vi "Choreo_Trajectory_GetTrajState.vi"(9 "index":i32, 11 "ChoreoTrajectory":T2) -> (3 "ChoreoTrajectoryState":T1)   [LabVIEW 2019, in "ChoreoLib.lvlib"]
doc: "Return a single trajectory state from the trajectory.\n\nInputs: \n - ChoreoTrajectory - cluster - Input trajectory\n - Index - integer - index into the trajectory state array. Beginning index is zero.\n\nOutputs:\n - Trajectory state - cluster - the selectred trajectory state.."
uses:
  ChoreoLib.lvlib
  TypeDef/ChoreoTrajectory.ctl
  TypeDef/ChoreoTrajectoryState.ctl
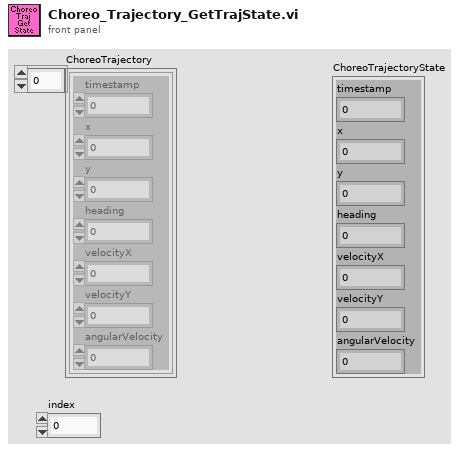
[diagram p1: front panel]
types:
  T1 = typedef "ChoreoLib.lvlib/ChoreoTrajectoryState.ctl" = cluster{"timestamp":dbl, "x":dbl, "y":dbl, "heading":dbl, "velocityX":dbl, "velocityY":dbl, "angularVelocity":dbl}
  T2 = typedef "ChoreoLib.lvlib/ChoreoTrajectory.ctl" = T1[]
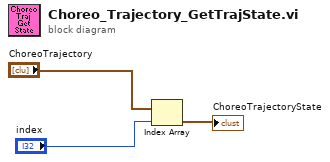
[diagram p0: block diagram]
diagram:
  n1 = Index Array(array="ChoreoTrajectory", index="index") -> (element=→"ChoreoTrajectoryState":T1)
